vi "Lissage.vi"() -> ()   [LabVIEW 2018]
panel:
  in  "stop":bool
  out "Graphe déroulant":cluster{dbl, dbl, dbl}(graph)
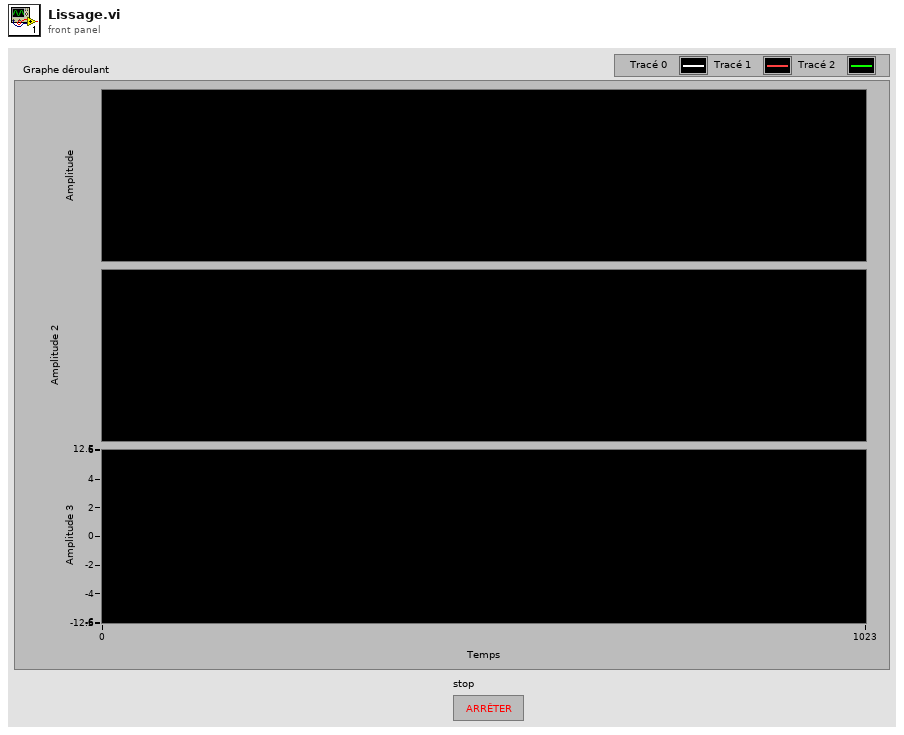
[diagram p1: front panel]
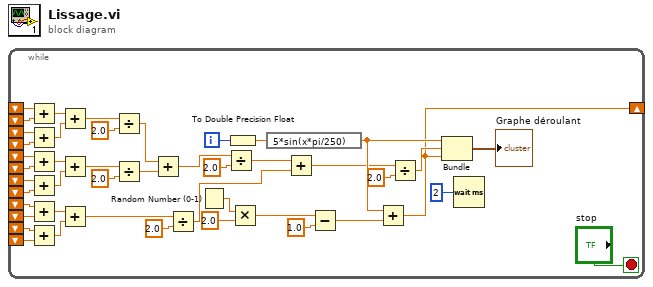
[diagram p0: block diagram]
diagram:
  n1 = while {
    shift-right: [w1] -> _
    shift-left: _ -> [w29]
    shift-left: _ -> [w30]
    shift-left: _ -> [w31]
    shift-left: _ -> [w32]
    shift-left: _ -> [w23]
    shift-left: _ -> [w22]
    shift-left: _ -> [w21]
    shift-left: _ -> [w20]
    shift-left: _ -> [w19]
    shift-left: _ -> [w18]
    shift-left: _ -> [w17]
    shift-left: _ -> [w16]
    i -> [w42]
    stop <- "stop" stop-if-true
    n2 = Add(x=w29, y=w30) -> (x+y=w34:dbl)
    n3 = Add(x=w31, y=w32) -> (x+y=w33:dbl)
    n4 = Add(x=w23, y=w22) -> (x+y=w27:dbl)
    n5 = Add(x=w21, y=w20) -> (x+y=w26:dbl)
    n6 = Add(x=w19, y=w18) -> (x+y=w25:dbl)
    n7 = Add(x=w17, y=w16) -> (x+y=w24:dbl)
    n8 = Add(x=w34, y=w33) -> (x+y=w13:dbl)
    n9 = Add(x=w27, y=w26) -> (x+y=w9:dbl)
    n10 = Add(x=w25, y=w24) -> (x+y=w11:dbl)
    n11 = Divide(x=w13, y=2.0) -> (x/y=w7:dbl)
    n12 = Divide(x=w9, y=2.0) -> (x/y=w6:dbl)
    n13 = Add(x=w7, y=w6) -> (x+y=w4:dbl)
    n14 = Divide(x=w11, y=2.0) -> (x/y=w2:dbl)
    n15 = Random Number (0-1)() -> (number: 0 to 1=w40:dbl)
    n16 = Divide(x=w4, y=2.0) -> (x/y=w3:dbl)
    n17 = To Double Precision Float(number=w42) -> (double precision float=w44:dbl)
    n18 = Multiply(x=w40, y=2.0) -> (x*y=w38:dbl)
    n19 = expression code="5*sin(x*pi/250)"(w44) -> (w36:dbl)
    n20 = Add(x=w3, y=w2) -> (x+y=w14:dbl)
    n21 = Subtract(x=w38, y=1.0) -> (x-y=w35:dbl)
    n22 = Add(x=w36, y=w35) -> (x+y=w1:dbl)
    n23 = Divide(x=w14, y=2.0) -> (x/y=w28:dbl)
    n24 = Bundle(w36, w28, w1) -> (→"Graphe déroulant":cluster{dbl, dbl, dbl})  [unwired: 1 in]
    n25 = Wait (ms)(milliseconds to wait=u32 2 ("attente (ms)")) -> ()  [unwired: 1 out]
  }
